vi "2025_day3.vi"() -> ()   [LabVIEW 2025]
uses:
  <userlib>/_OpenG.lib/string/string.llb/openg_string.lvlib
panel:
  out "Task 2 - Total output joltage":u64
  out "Task 1 - Total output joltage":i32
  in  "Switch":bool caption="Ex. Data  vs.  User Data"
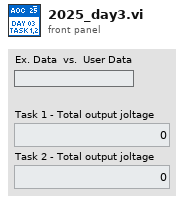
[diagram p1: front panel]
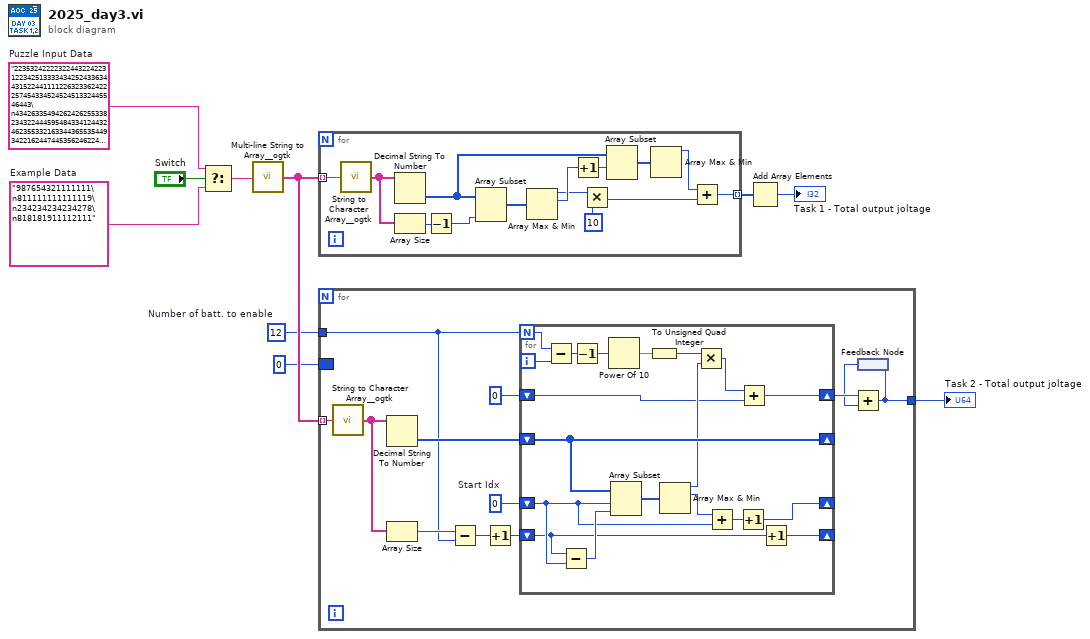
[diagram p0: block diagram]
diagram:
  w3 = 12  # Number of batt. to enable
  w8 = "2235324222232244322422312234251333343425243363443152244111122632336242225745433452452451332445546443\n4342633549426242625533823432244459548433412443246235533216334436553544934221624474453562462242374424\n8434422643334243334243543423324744383442433444345133334323443723387546342444334386334543315426294343\n3314333333333253227333289433334173324336435282333332374344333346362333436223333531247332233332431333\n2432233222232224244344214455331424832252285224272831524326258455142222732648222482237235275222221622\n64565555346465655641734596543544465466743454564325764433365445644656237935363655634948443435862..."  # Puzzle Input Data
  w9 = "987654321111111\n811111111111119\n234234234234278\n818181911112111"  # Example Data
  n1 = Select(t=w8, s="Switch", f=w9) -> (s? t:f=w7:string)
  n2 = call <userlib>:"Multi-line String to Array__ogtk.vi"("string"=w7) -> ("lines"=w4:string[])
  n3 = for {
    tunnel: w4 -> [w24] mode=indexing
    tunnel: [w11] -> w6 mode=indexing
    n4 = call <userlib>:"String to Character Array__ogtk.vi"("Input String"=w24) -> ("Character Array"=w23:string[])
    n5 = Decimal String To Number(string=w23) -> (number=w18:i32[])  [unwired: 2 in, 1 out]
    n6 = Array Size(array=w23) -> (size(s)=w22:i32)
    n7 = Decrement(x=w22) -> (x-1=w21:i32)
    n8 = Array Subset(array=w18, length=w21) -> (w20:i32[])  [unwired: 1 in]
    n9 = Array Max & Min(array=w20) -> (max value=w15:i32, max index (indices)=w19:i32)  [unwired: 2 out]
    n10 = Increment(x=w19) -> (x+1=w17:i32)
    n11 = Multiply(x=w15, y=10) -> (x*y=w12:i32)
    n12 = Array Subset(array=w18, index=w17) -> (w16:i32[])  [unwired: 1 in]
    n13 = Array Max & Min(array=w16) -> (max value=w13:i32)  [unwired: 3 out]
    n14 = Add(x=w13, y=w12) -> (x+y=w11:i32)
  }
  n15 = for {
    tunnel: w4 -> [w36] mode=indexing
    tunnel: w3 -> [w29]
    border: u64 0 -> [_]
    tunnel: [w25] -> w2
    w31 = 0  # Start Idx
    n16 = call <userlib>:"String to Character Array__ogtk.vi"("Input String"=w36) -> ("Character Array"=w35:string[])
    n17 = Decimal String To Number(string=w35) -> (number=w33:i32[])  [unwired: 2 in, 1 out]
    n18 = Array Size(array=w35) -> (size(s)=w34:i32)
    n19 = Subtract(x=w34, y=w29) -> (x-y=w32:i32)
    n20 = Increment(x=w32) -> (x+1=w30:i32)
    n21 = for {
      N: w29 -> [w45]
      shift-right: [w54] -> _
      shift-left: w33 -> [w54]
      shift-right: [w47] -> _
      shift-left: w30 -> [w48]
      shift-right: [w49] -> _
      shift-left: w31 -> [w51]
      shift-right: [w40] -> w27
      shift-left: u64 0 -> [w39]
      i -> [w46]
      n22 = Subtract(x=w45, y=w46) -> (x-y=w44:i32)
      n23 = Subtract(x=w48, y=w51) -> (x-y=w55:i32)
      n24 = Decrement(x=w44) -> (x-1=w37:i32)
      n25 = Power Of 10(x=w37) -> (10^x=w43:dbl)
      n26 = Array Subset(array=w54, index=w51, length=w55) -> (w53:i32[])
      n27 = To Unsigned Quad Integer(1:w43) -> (0:w42:u64)
      n28 = Array Max & Min(array=w53) -> (max value=w41:i32, max index (indices)=w52:i32)  [unwired: 2 out]
      n29 = Multiply(x=w42, y=w41) -> (x*y=w38:u64)
      n30 = Add(x=w52, y=w51) -> (x+y=w50:i32)
      n31 = Increment(x=w50) -> (x+1=w49:i32)
      n32 = Add(x=w38, y=w39) -> (x+y=w40:u64)
      n33 = Increment(x=w48) -> (x+1=w47:i32)
    }
    n34 = feedback #1() -> (w26:u64)
    n35 = Add(x=w27, y=w26) -> (x+y=w25:u64)
    n36 = feedback-in #1(w25) -> ()
  }
  "Task 2 - Total output joltage" <- w2
  n37 = Add Array Elements(numeric array=w6) -> (sum=→"Task 1 - Total output joltage":i32)
